vi "Stop Trial.vi"(8 "error in (no error)":errorcluster, 10 "Stop Acquiring":bool, 11 "Accelerometer in":refnum<class "Accelerometer.lvclass">) -> (0 "error out":errorcluster, 3 "Accelerometer out":refnum<class "Accelerometer.lvclass">)   [LabVIEW 2020, in "Accelerometer.lvlib" / "Accelerometer.lvclass"]
uses:
  Accelerometer.lvclass
  Accelerometer.lvclass/Accelerometer.ctl
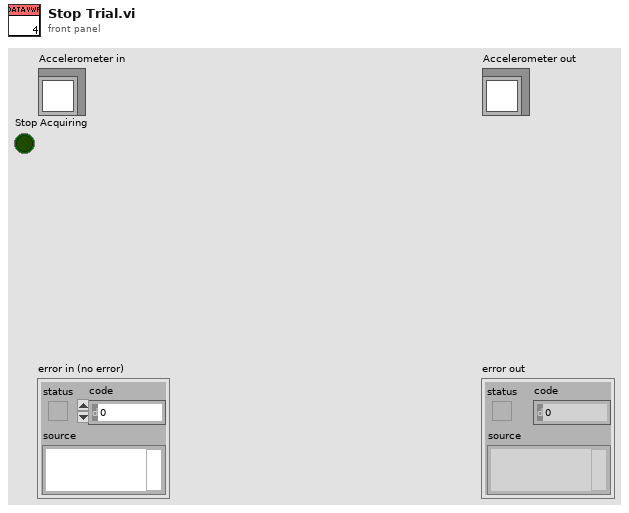
[diagram p1: front panel]
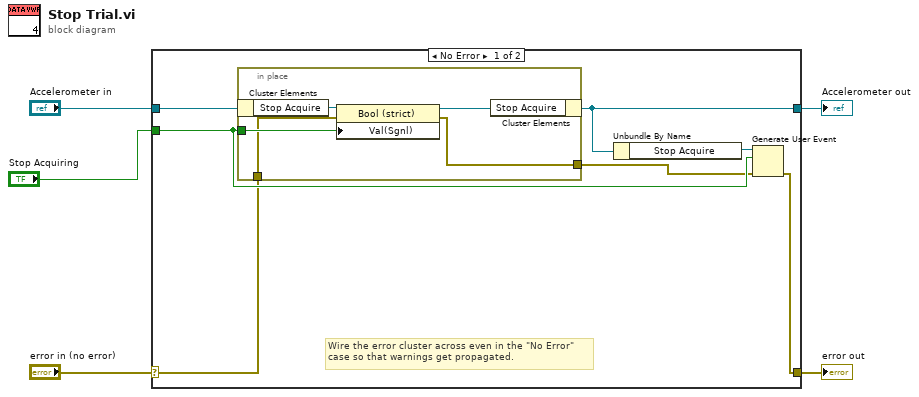
[diagram p0: block diagram]
diagram:
  n1 = case shown="No Error" "error in (no error)" {
    selector: "error in (no error)" -> [w8 w19]
    tunnel: [w6 w19] -> w4
    tunnel: [w11 w18] -> w2
    tunnel: "Accelerometer in" -> [w12 w18]
    tunnel: "Stop Acquiring" -> [w9 _]
    frame No Error {
      # "Wire the error cluster across even in the \"No Error\"\ncase so that warnings get propagated."
      n2 = in-place {
        in-place-border: w9 -> [w15]
        in-place-border: w8 -> [w14]
        in-place-border: [w13] -> w7
        n3 = in-place-cluster #1(w12) -> ("Stop Acquire"=w17:refnum<vi>)
        n4 = property class="Bool (strict)"(reference=w17, error in=w14, "Val(Sgnl)"=w15) -> (reference out=w16:refnum<vi>, error out=w13:errorcluster)
        n5 = in-place-cluster #1("Stop Acquire"=w16) -> (w11:refnum<class "Accelerometer.lvclass">)
      }
      n6 = Unbundle By Name(w11) -> ("Stop Acquire"=w10:refnum<user-event>)
      n7 = Generate User Event(user event=w10, event data cluster=w9, error in=w7) -> (error out=w6:errorcluster)  [unwired: 1 in, 1 out]
    }
    frame Error {
    }
  }
  "error out" <- w4
  "Accelerometer out" <- w2
